vi "Define If Not.vi"(9 "token string":string, 11 "String in":string) -> (3 "String out":string)   [LabVIEW 2014, in "C Header Generator.lvlib"]
uses:
  C Header Generator.lvlib
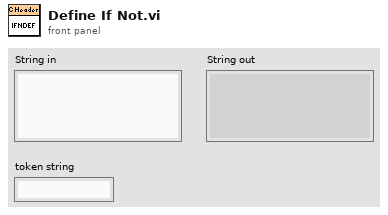
[diagram p1: front panel]
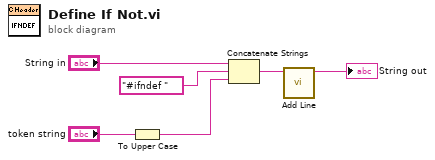
[diagram p0: block diagram]
diagram:
  n1 = To Upper Case(1:"token string") -> (0:w1:string)
  n2 = Concatenate Strings("String in", "#ifndef ", w1) -> (w3:string)
  n3 = call "Add Line.vi"("String in"=w3) -> ("String out"=→"String out":string)  [unwired: 10 in]
